vi "Raw Data Start Transfer.vi"(7 "Command string":string, 8 "error in (no error)":errorcluster, 9 "#pts string":string, 10 "Network Info":T1 {"Last Comm Time" format="%<%H:%M:%S%3u\n%Y/%m/%d>T"; "Remote Port" format="%.0x"}, 11 "Refnum in":T3) -> (0 "error out":errorcluster, 3 "Network Info Out":T1 {"Last Comm Time" format="%<%H:%M:%S%3u\n%Y/%m/%d>T"; "Remote Port" format="%.0x"})   [LabVIEW 2023]
doc: "Author: Scott Hannahs <sth@magnet.fsu.edu>\nCopyright 2018 Florida State University, All rights reserved."
uses:
  RT Controls/FPGA SCH Digitizer Ref.ctl
  RT Controls/Network Info.ctl
  RT Controls/RT System Auth Level.ctl
  RT Host Globals.vi
  TCP Functions/TCP Write Length and Data (STR).vi
  TCP Functions/TCP Write Length and Data (U32).vi
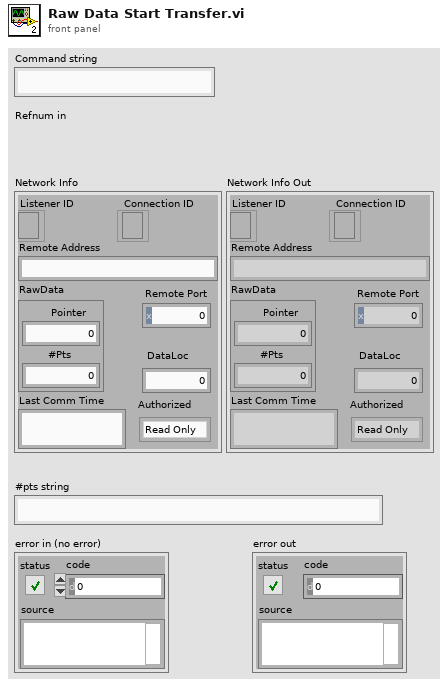
[diagram p1: front panel]
types:
  T1 = typedef "Network Info.ctl" = cluster{"Listener ID":refnum<k5>, "Connection ID":refnum<k5>, "Remote Address":string, "Remote Port":u16, "DataLoc":u32, "RawData":cluster{"#Pts":u32, "Pointer":u32}, "Last Comm Time":timestamp, "Authorized":T2}
  T2 = typedef "RT System Auth Level.ctl" = enum16{"Read Only", "Operator", "Admin"}
  T3 = typedef "FPGA SCH Digitizer Ref.ctl" = refnum<k20>
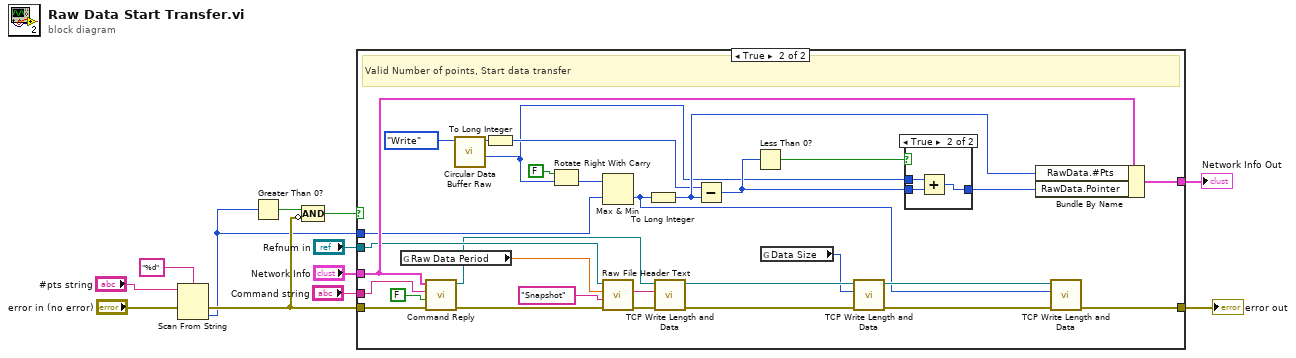
[diagram p0: block diagram]
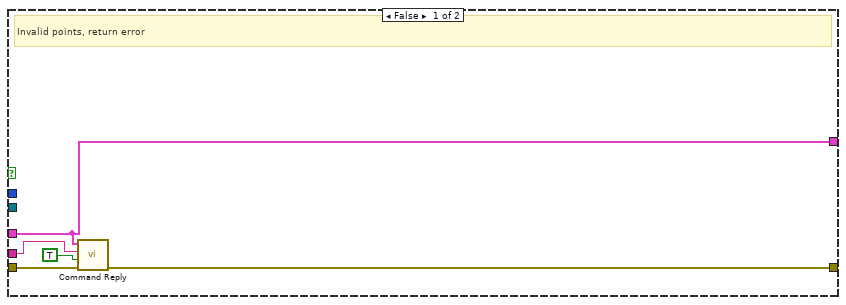
[diagram p2: hidden frame]
diagram:
  n1 = Scan From String(format string="%d", input string="#pts string", error in="error in (no error)") -> (error out=w9:errorcluster, output 1=w8:i32)  [unwired: 2 in, 2 out]
  n2 = Greater Than 0?(x=w8) -> (x > 0?=w10:bool)
  n3 = Compound Arithmetic op=AND(w10, invert w9) -> (w11:bool)
  n4 = case shown="True" w11 {
    tunnel: [w14 w33] -> w3
    tunnel: "Network Info" -> [w13 w37]
    tunnel: "Command string" -> [w15 w36]
    tunnel: w8 -> [_ w35]
    tunnel: w9 -> [w16 w34]
    tunnel: "Refnum in" -> [_ w32]
    tunnel: [w13 w21] -> w1
    frame False {
      # "Invalid points, return error"
      n5 = call "Command Reply.vi"("Error In"=w16, "Error?"=TRUE, "String"=w15, "Network Info"=w13) -> ("error out"=w14:errorcluster)  [unwired: 6 in, 1 out]
    }
    frame True {
      # "Valid Number of points, Start data transfer"
      n6 = global read "RT Host Globals.vi" "Raw Data Period"() -> (w31:dbl)
      n7 = call "Command Reply.vi"("Error In"=w34, "Error?"=FALSE, "String"=w36, "Network Info"=w37) -> ("error out"=w30:errorcluster, "TCP Network Connection out"=w28:refnum<k5>)  [unwired: 6 in]
      n8 = call "Circular Data Buffer Raw.vi"("Enum"=enum16{"Initialize", "Write", "Read", "Clear"}."Write") -> ("Buffer Size"=w18:u32, "Next Write"=w20:u32)  [unwired: 8 in, 1 out]
      n9 = To Long Integer(number=w20) -> (32bit integer=w42:i32)
      n10 = Rotate Right With Carry(2:w18, 3:FALSE ("carry")) -> (0:w38:u32)  [unwired: 1 out]
      n11 = Max & Min(x=w38, y=w35) -> (min(x,y)=w23:u32)  [unwired: 1 out]
      n12 = call "Raw File Header Text.vi"("error in (no error)"=w30, "Type"="Snapshot", "Raw Data Period"=w31, "FPGA Refnum out"=w32) -> ("error out"=w26:errorcluster, "concatenated string"=w25:string)  [unwired: 5 in, 1 out]
      n13 = To Long Integer(number=w23) -> (32bit integer=w46:i32)
      n14 = call-poly "TCP Write Length and Data.vi"("Error In"=w26, "Data"=w25, "connection ID"=w28) -> ("Error Out"=w27:errorcluster, "connection ID out"=w29:refnum<k5>)  [unwired: 7 in]
      n15 = Subtract(x=w42, y=w46) -> (x-y=w40:i32)
      n16 = Less Than 0?(x=w40) -> (x < 0?=w39:bool)
      n17 = global read "RT Host Globals.vi" "Data Size"() -> (w24:u32)
      n18 = call-poly "TCP Write Length and Data.vi"("Error In"=w27, "Data"=w24, "connection ID"=w29) -> ("Error Out"=w44:errorcluster, "connection ID out"=w45:refnum<k5>)  [unwired: 7 in]
      n19 = case shown="True" w39 {
        tunnel: w40 -> [w48 w51]
        tunnel: w18 -> [_ w50]
        tunnel: [w48 w49] -> w41
        frame False {
        }
        frame True {
          n20 = Add(x=w50, y=w51) -> (x+y=w49:u32)
        }
      }
      n21 = Bundle By Name(cluster=w37, "RawData.#Pts"=w46, "RawData.Pointer"=w41) -> (w21:T1)
      n22 = call-poly "TCP Write Length and Data.vi"("Error In"=w44, "Data"=w23, "connection ID"=w45) -> ("Error Out"=w33:errorcluster)  [unwired: 7 in, 1 out]
    }
  }
  "error out" <- w3
  "Network Info Out" <- w1
